vi "Deconstruct PDU.vi"(8 "error in (no error)":errorcluster, 11 "modbus data unit in":refnum<class "ELAN PDU.lvclass">) -> (0 "error out":errorcluster, 1 "command":cluster{"type":string, "number":u8}={"type"="k", "number"=1}, 2 "channel state":T1, 3 "collective state":u8, 4 "data":u8[](array[numeric]), 5 "source address":u8, 7 "target address":u8)   [LabVIEW 2021, in "ELAN PDU.lvclass"]
uses:
  ELAN PDU.lvclass
  Elan channel state.ctl
  ELAN PDU.lvclass/ELAN PDU.ctl
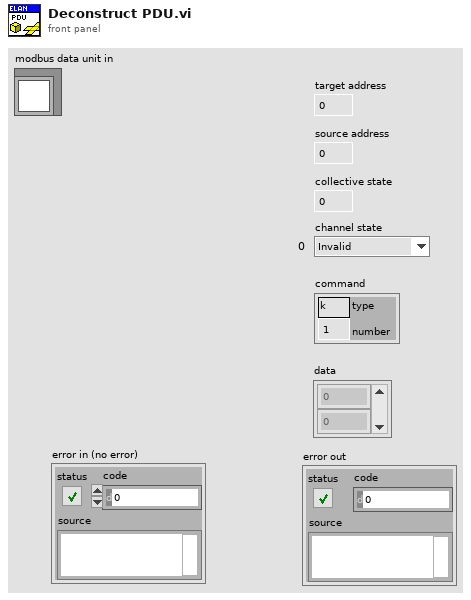
[diagram p1: front panel]
types:
  T1 = typedef "ELAN PDU.lvclass/Elan channel state.ctl" = enum16{"Invalid", "Warm-up", "Pause", "Standby", "Measure", "Zero calibration", "Adjust component slope", "Not yet defined1", "Adjust curve dip", "Adjust linearization sensitivity", "Adjust temperature compensation", "Adjust pressure compensation", "Adjust linearization zero", "Not yet defined2", "Autocal", "Adjust phase", "Zero calibration of O2 sensor", "Synchronous zero calibration", "Purging for synchronous zero calibration", "Adjust analog output", "Adjust analog input", "Autocal check"}
  T2 = typedef "ELAN PC PDU.lvclass/Elan channel state.ctl" = enum16{"Invalid", "Warm-up", "Pause", "Standby", "Measure", "Zero calibration", "Adjust component slope", "Not yet defined1", "Adjust curve dip", "Adjust linearization sensitivity", "Adjust temperature compensation", "Adjust pressure compensation", "Adjust linearization zero", "Not yet defined2", "Autocal", "Adjust phase", "Zero calibration of O2 sensor", "Synchronous zero calibration", "Purging for synchronous zero calibration", "Adjust analog output", "Adjust analog input", "Autocal check"}
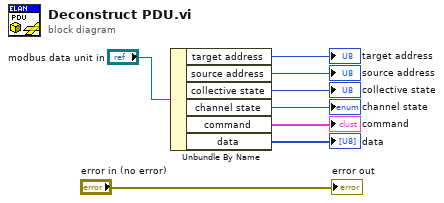
[diagram p0: block diagram]
diagram:
  n1 = Unbundle By Name("modbus data unit in") -> ("target address"=→"target address":u8, "source address"=→"source address":u8, "collective state"=→"collective state":u8, "channel state"=→"channel state":T2, "command"=→"command":cluster{"type":string, "number":u8}, "data"=→"data":u8[])
  "error out" <- "error in (no error)"
